vi "HAL camera program for acquisition - SubVI.vi"(2 "error in":errorcluster, 3 "Camera Parameters (important)":T1 {"Shutter" items=["Auto", "Stay Open", "Always Closed"]; "Readout Settings"."Trigger Mode" items=["Internal", "External"]; "EM CCD Gain" scale=0.01..255.0; "Exposure Time (sec)" scale=0.001..10.0 scale format="%#_1g"}) -> (0 "error out":errorcluster, 1 "Actual Exposure Time (sec)":sgl)   [LabVIEW 2014]
uses:
  HAL camera parameters important 1 - SubVI.ctl
  ixon readout settings - SubVI.ctl
  andor acquisition mode.ctl
  image size - SubVI.ctl
  camera globals - SubVI.vi
panel:
  # "Camera: Andor iXon"
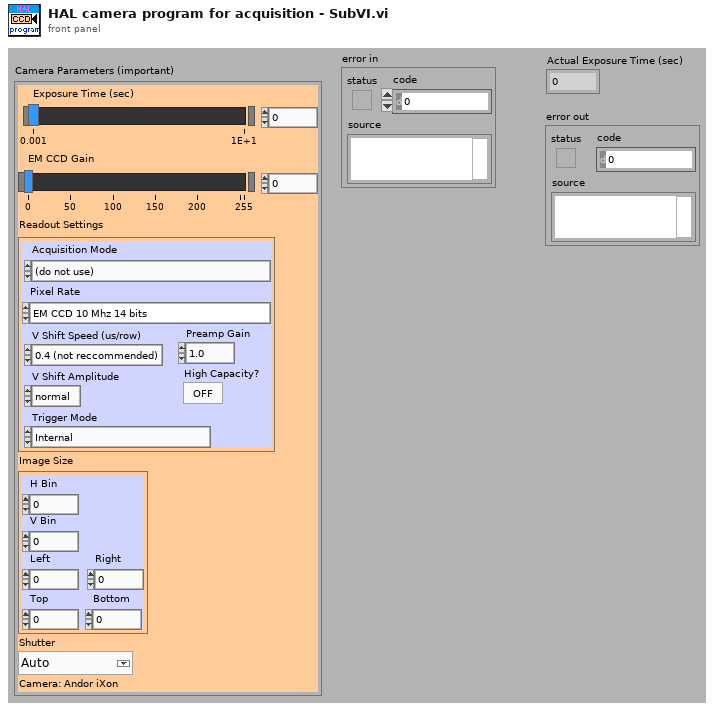
[diagram p1: front panel]
types:
  T1 = typedef "HAL camera parameters important 1 - SubVI.ctl" = cluster{"Exposure Time (sec)":sgl, "EM CCD Gain":u8, "Readout Settings":T2, "Image Size":T4, "Shutter":i32}
  T2 = typedef "ixon readout settings - SubVI.ctl" = cluster{"Acquisition Mode":T3, "Pixel Rate":enum16{"EM CCD 10 Mhz 14 bits", "EM CCD 5 Mhz 14 bits", "EM CCD 3 Mhz 14 bits", "EM CCD 1 Mhz 16 bits", "Standard CCD 3 Mhz 14 bits", "Standard CCD 1 Mhz 16 bits"}, "High Capacity?":bool, "V Shift Speed (us/row)":enum16{"0.4 (not reccommended)", "0.6  (not reccommended)", "1.0  (not reccommended)", "1.8  (not reccommended)", "3.4  (not reccommended)", "6.6", "13.0"}, "V Shift Amplitude":enum16{"normal", "+1", "+2", "+3", "+4"}, "Preamp Gain":enum16{"1.0", "2.6"}, "Trigger Mode":u32}
  T3 = typedef "andor acquisition mode.ctl" = enum16{"(do not use)", "Single Scan", "Accumulate", "Kinetics", "Fast Kinetics", "Kinetics Run till Abort", "Frame Transfer", "Frame Transfer Run till Abort", "(do not use) ", "Time Delayed Integration"}
  T4 = typedef "image size - SubVI.ctl" = cluster{"H Bin":i32, "V Bin":i32, "Left":i32, "Top":i32, "Right":i32, "Bottom":i32}
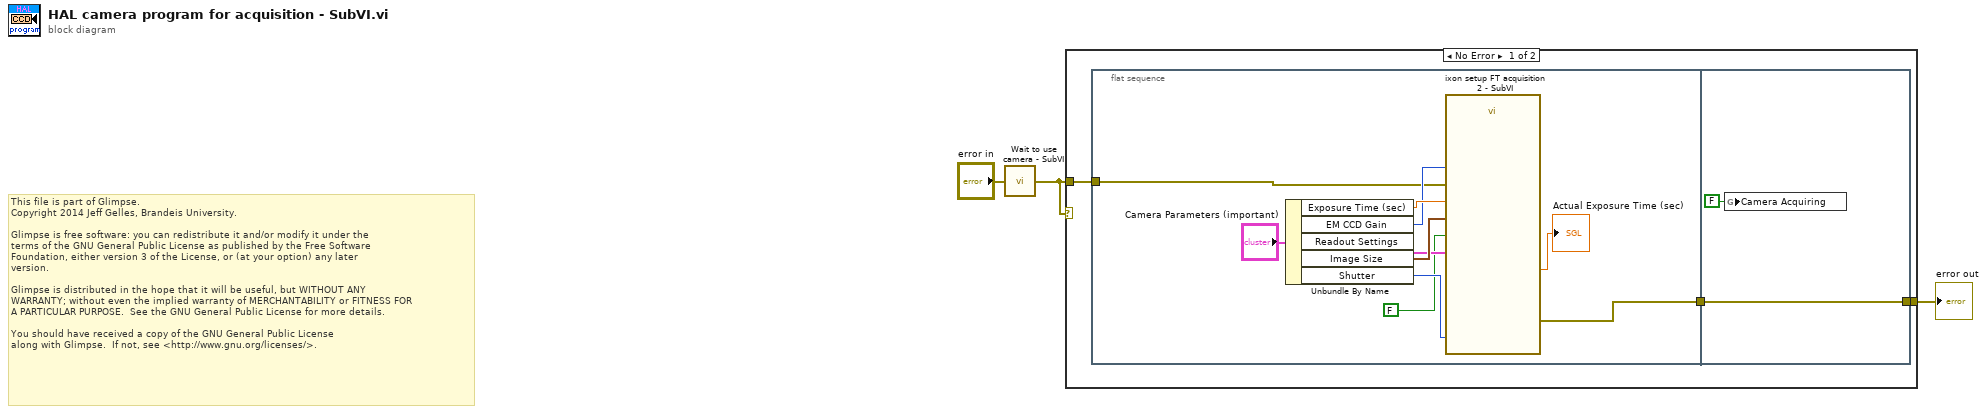
[diagram p0: block diagram]
diagram:
  # "This file is part of Glimpse. \nCopyright 2014 Jeff Gelles, Brandeis University.    \n\nGlimpse is free software: you can redistribute it and/or modify it under the \nterms of the GNU General Public License as published by the Free Software \nFoundation, either version 3 of the License, or (at your option) any later \nversion.\n\nGlimpse is distributed in the hope that it will be useful, but WITHOUT ANY \nWARRANTY; without even the implied warranty of MERCHANTABILITY or FITNESS FOR \nA PARTICULAR PURPOSE.  See the GNU General Public License for more details.\n\nYou should have received a copy of the GNU General Public License\nalong with Glimpse.  If not, see <http://www.gnu.org/licenses/>."
  n1 = call "Wait to use camera - SubVI.vi"("error in"="error in") -> ("error out"=w1:errorcluster)
  n2 = case shown="No Error" w1 {
    tunnel: [w6 w19] -> w3
    tunnel: w1 -> [w5 w19]
    frame No Error {
      n3 = flat-sequence {
        tunnel: w5 -> [w7]
        tunnel: [w16] -> w4
        tunnel: [w18] -> w6
        tunnel: w4 -> [w18]
        frame #0 {
          n4 = Unbundle By Name("Camera Parameters (important)") -> ("Exposure Time (sec)"=w13:sgl, "EM CCD Gain"=w10:u8, "Readout Settings"=w11:T2, "Image Size"=w12:T4, "Shutter"=w14:i32)
          n5 = call "ixon setup FT acquisition 2 - SubVI.vi"("Shutter"=w14, "EM CCD Gain"=w10, "Interactive?"=FALSE, "error in (no error)"=w7, "Exposure Time (sec)"=w13, "Readout Settings"=w11, "Image Size"=w12) -> ("error out"=w16:errorcluster, "Actual Exposure Time (sec)"=→"Actual Exposure Time (sec)":sgl)  [unwired: 1 in, 2 out]
        }
        frame #1 {
          n6 = global write "camera globals - SubVI.vi" "Camera Acquiring"(FALSE ("Andor Aquiring")) -> ()
        }
      }
    }
    frame Error {
    }
  }
  "error out" <- w3
